vi "Periodic Tasks.vi"(8 "error in":errorcluster) -> (3 "Boolean":bool)   [LabVIEW 2020]
doc: "This VI runs in parallel to other tasks. It can contain as many user-defined periodic loops as you need. These can carry out PID or other sorts of timed response."
uses:
  Utility/Global_STOP.vi
  Systems/SwerveDrive/SwerveDrive_ACT.lvlib
  Systems/Game Controller/GameController_SEN.lvlib
  Systems/PigeonIMU/PigeonIMU_SEN.lvlib
  Systems/NTV Read Write/NTV Read Write.lvlib
  Systems/Arm/Arm_ACT.lvlib
  Systems/Extention/Extend_ACT.lvlib
  Systems/Wrist/Wrist_ACT.lvlib
  Systems/Sholder/Sholder_ACT.lvlib
  Systems/MotionMaser/MotionMaster_SubCMD.lvlib
  Systems/Grabber/Grabber_ACT.lvlib
  Systems/AUTO 2023/2023-Auto_CMD.lvlib
  Systems/SwerveOdometry/Swerve_Odometry_SEN.lvlib
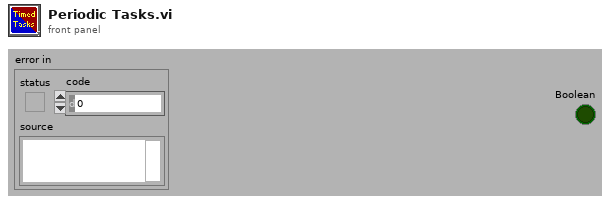
[diagram p1: front panel]
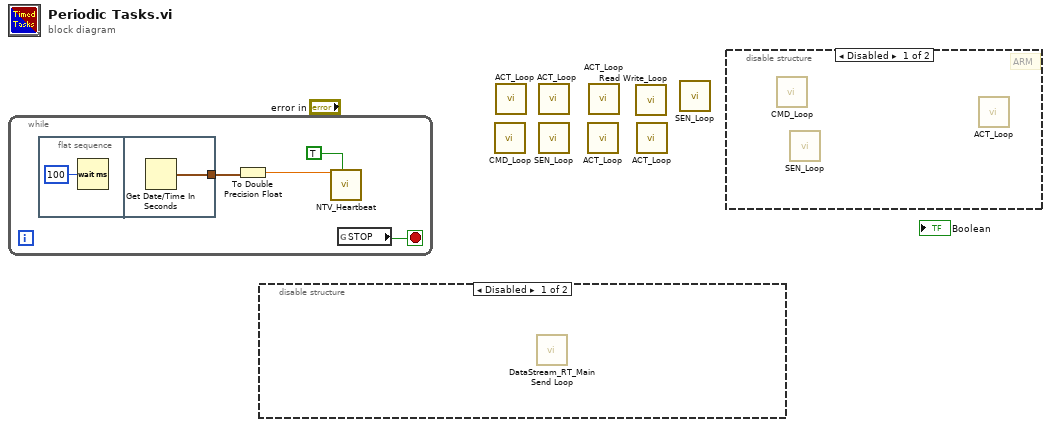
[diagram p0: block diagram]
diagram:
  n1 = while {
    stop <- w4 stop-if-true
    n2 = flat-sequence {
      tunnel: [w6] -> w2
      frame #0 {
        n3 = Wait (ms)(milliseconds to wait=u32 100) -> ()  [unwired: 1 out]
      }
      frame #1 {
        n4 = Get Date/Time In Seconds() -> (seconds since 1Jan1904=w6:timestamp)
      }
    }
    n5 = To Double Precision Float(number=w2) -> (double precision float=w1:dbl)
    n6 = call "NTV_Heartbeat.vi"("Read(f) Write(t)"=TRUE, "Heartbeat"=w1) -> ()  [unwired: 9 in, 1 out]
    n7 = global read "Global_STOP.vi" "STOP"() -> (w4:bool)
  }
  n8 = disable-structure shown="Disabled" {
    frame Disabled {
      n9 = call "DataStream_RT_Main Send Loop.vi"() -> ()  [unwired: 12 in]
    }
    frame Enabled {
    }
  }
  n10 = call "CMD_Loop.vi"() -> ()  [unwired: 12 in]
  n11 = call "ACT_Loop.vi"() -> ()  [unwired: 12 in]
  n12 = call "ACT_Loop.vi"() -> ()  [unwired: 12 in]
  n13 = call "SEN_Loop.vi"() -> ()  [unwired: 12 in]
  n14 = call "ACT_Loop.vi"() -> ()  [unwired: 12 in]
  n15 = call "ACT_Loop.vi"() -> ()  [unwired: 12 in]
  n16 = call "Read Write_Loop.vi"() -> ()  [unwired: 12 in]
  n17 = call "ACT_Loop.vi"() -> ()  [unwired: 12 in]
  n18 = call "SEN_Loop.vi"() -> ()  [unwired: 12 in]
  n19 = disable-structure shown="Disabled" {
    frame Disabled {
      # "ARM"
      n20 = call "CMD_Loop.vi"() -> ()  [unwired: 12 in]
      n21 = call "SEN_Loop.vi"() -> ()  [unwired: 12 in]
      n22 = call "ACT_Loop.vi"() -> ()  [unwired: 12 in]
    }
    frame Enabled {
    }
  }
